vi "NIDCPower_channel_ganging - delete advanced sequence.vi"(8 "error in (no error)":errorcluster, 10 "sequence name":string="SourceVoltages", 11 "Ganged Session In":T1) -> (0 "error out":errorcluster, 3 "Ganged Session Out":T1)   [LabVIEW 2021]
uses:
  ctl/NIDCPower_channel_ganging - ctl - ganged session.ctl
  ctl/NIDCPower_channel_ganging - ctl - ganged config.ctl
  ctl/NIDCPower_channel_ganging - ctl - channel mode.ctl
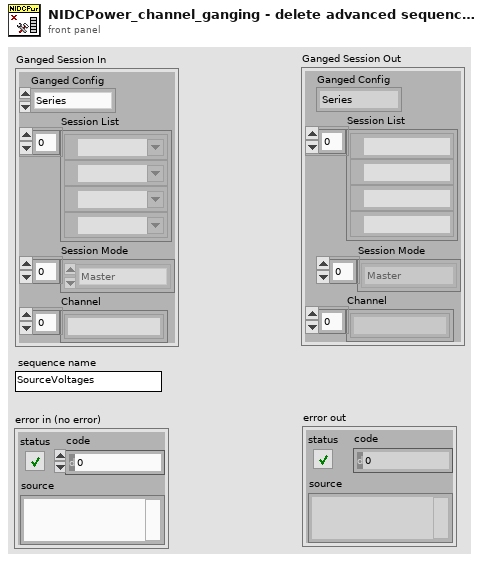
[diagram p1: front panel]
types:
  T1 = typedef "NIDCPower_channel_ganging - ctl - ganged session.ctl" = cluster{"Ganged Config":T2, "Session List":refnum<k15>[], "Session Mode":T3[], "Channel":string[]}
  T2 = typedef "NIDCPower_channel_ganging - ctl - ganged config.ctl" = enum32{"Series", "Parallel", "Manual"}
  T3 = typedef "NIDCPower_channel_ganging - ctl - channel mode.ctl" = enum32{"Master", "Slave", "Slave - Inverted"}
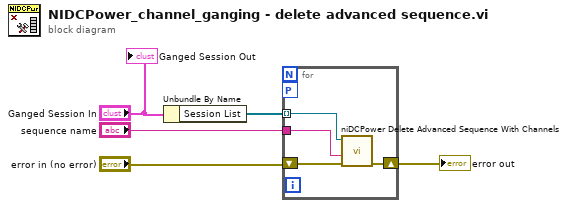
[diagram p0: block diagram]
diagram:
  n1 = Unbundle By Name("Ganged Session In") -> ("Session List"=w3:refnum<k15>[])
  n2 = for {
    tunnel: "sequence name" -> [w9]
    tunnel: w3 -> [w8] mode=indexing
    shift-right: [w6] -> w5
    shift-left: "error in (no error)" -> [w7]
    workers-P: _ -> [_]
    n3 = call <instrlib>:"niDCPower Delete Advanced Sequence With Channels.vi"("error in (no error)"=w7, "sequence name"=w9, "instrument handle"=w8) -> ("error out"=w6:errorcluster)  [unwired: 7 in, 1 out]
  }
  "error out" <- w5
  "Ganged Session Out" <- "Ganged Session In"
